vi "plotAnkleTraj.vi"(4 "AnkleTraj_Prev":dbl[][](array[numeric]), 5 "AnkleTraj_history":dbl[][](array[numeric]), 6 "Init?":bool, 8 "error in (no error)":errorcluster, 9 "PreviousPlotNum":i32, 10 "3D graph in":refnum<k7>) -> (0 "error out":errorcluster, 1 "LastPlotNum":i32=1, 2 "3D graph out":refnum<k7>)   [LabVIEW 2016]
uses:
  <vilib>/Platform/NI_3dgraph.lvlib
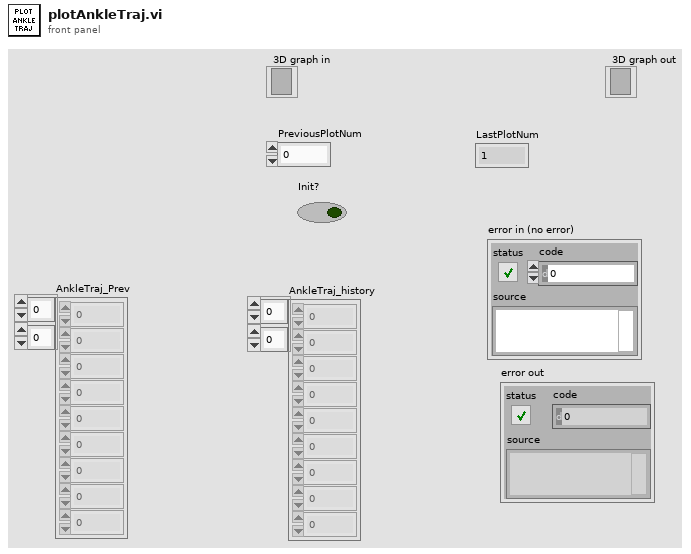
[diagram p1: front panel]
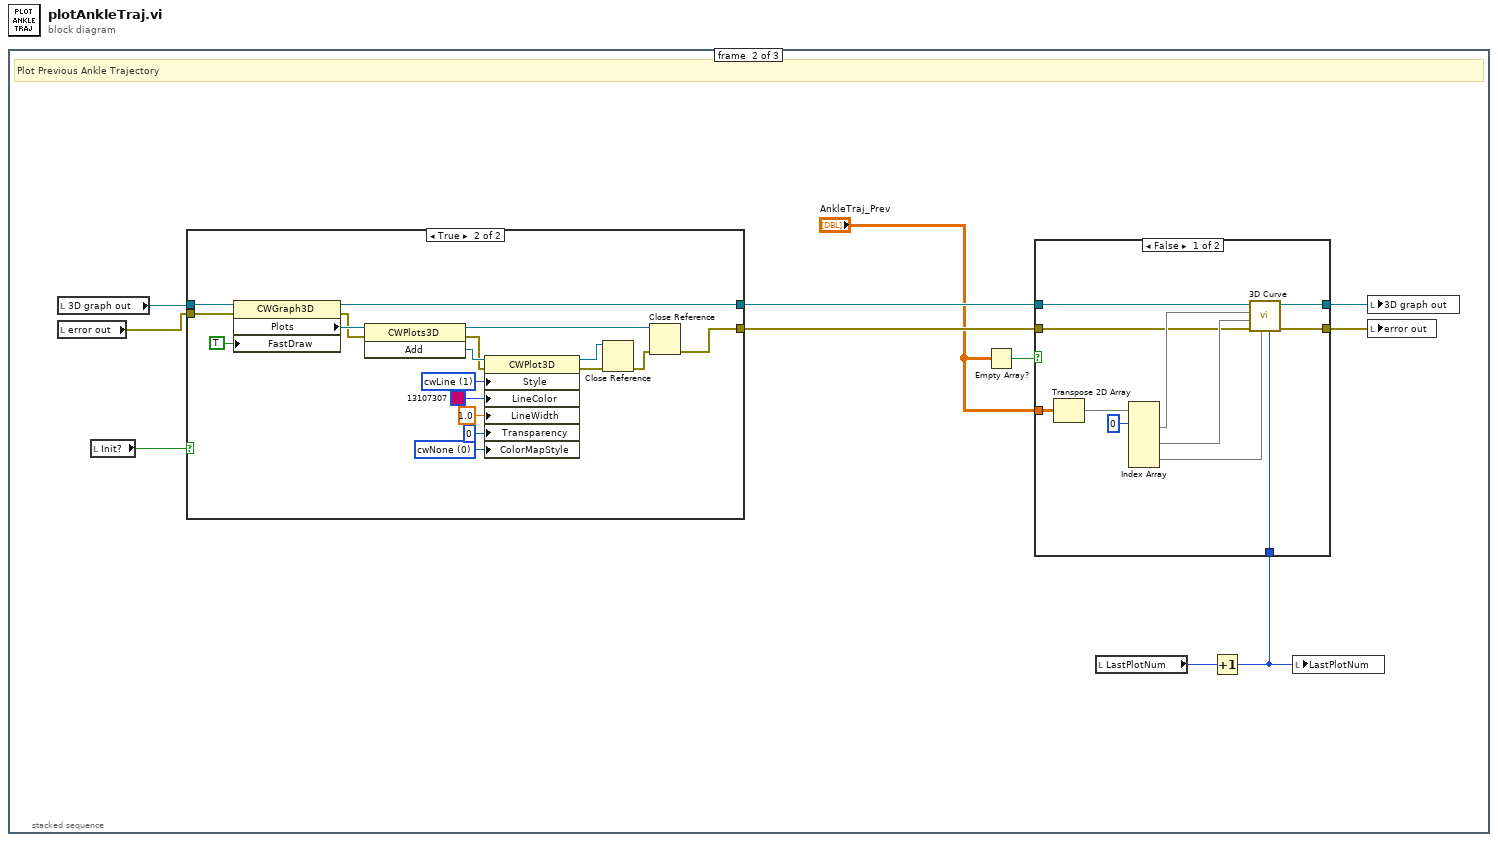
[diagram p0: block diagram]
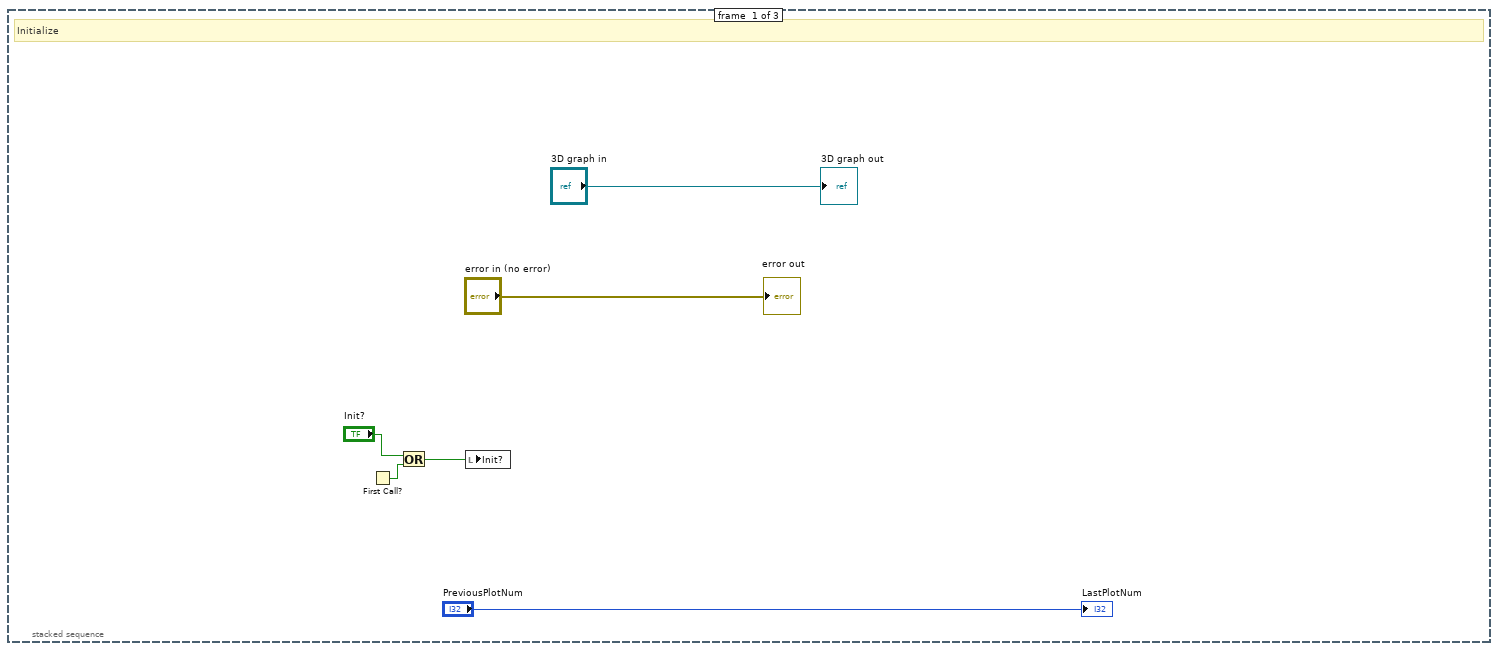
[diagram p2: hidden frame]
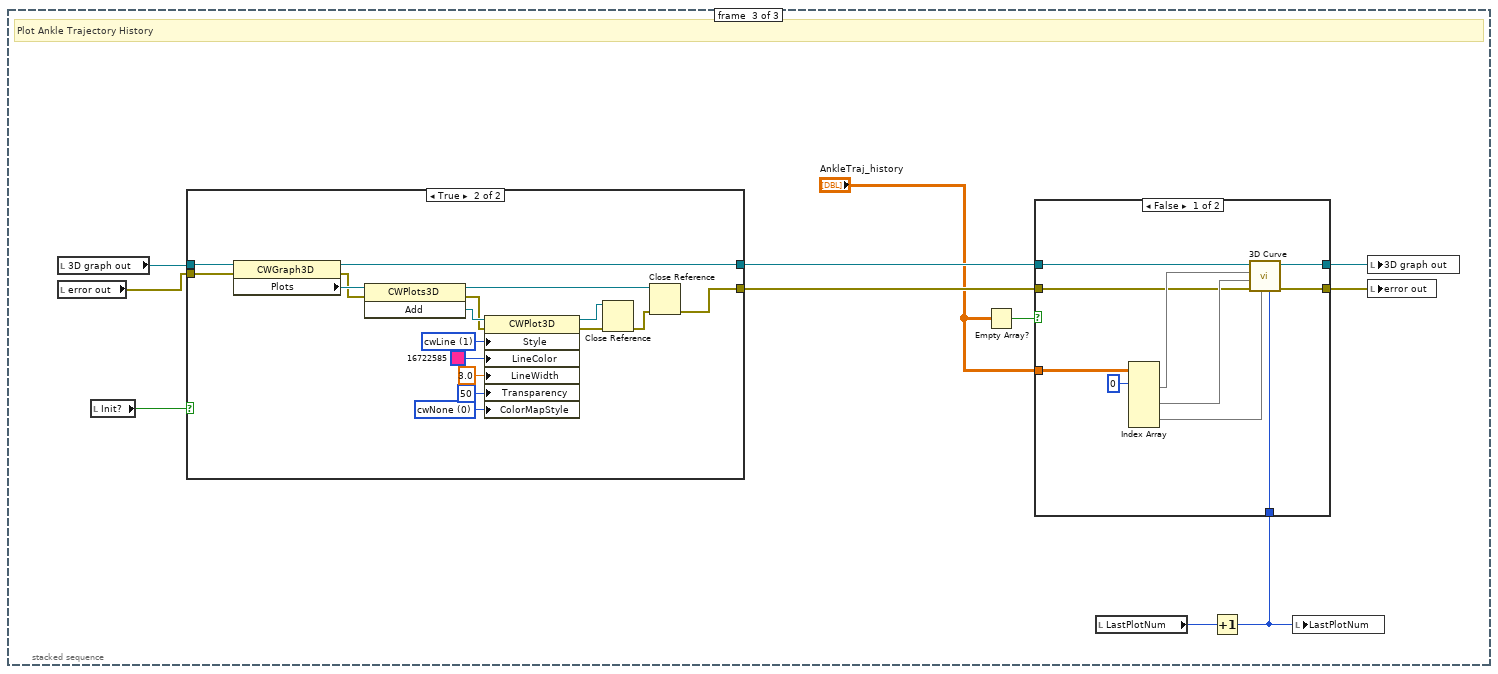
[diagram p5: hidden frame]
diagram:
  n1 = stacked-sequence {
    frame #0 {
      # "Initialize"
      n2 = First Call?() -> (First Call?: T/F=w3:bool)
      n3 = Or(x="Init?", y=w3) -> (x .or. y?=w1:bool)
      n4 = local write "Init?"(w1) -> ()
      "LastPlotNum" <- "PreviousPlotNum"
      "error out" <- "error in (no error)"
      "3D graph out" <- "3D graph in"
    }
    frame #1 {
      # "Plot Previous Ankle Trajectory"
      n5 = local read "3D graph out"() -> (w9:refnum<k7>)
      n6 = local read "error out"() -> (w8:errorcluster)
      n7 = local read "Init?"() -> (w7:bool)
      n8 = case shown="True" w7 {
        tunnel: w8 -> [w31 w43]
        tunnel: w9 -> [w32 w40]
        tunnel: [w32 w39] -> w17
        tunnel: [w31 w34] -> w16
        frame False {
        }
        frame True {
          w37 = 0 items=["cwNone", "cwShaded", "cwColorSpectrum", "cwGrayScale", "cwCustom"] ("ColorMapStyle")
          w50 = 1 items=["cwLine"=1, "cwPoint"=2, "cwLinePoint"=3, "cwHiddenLine"=4, "cwSurface"=5, "cwSurfaceLine"=6, "cwSurfaceNormal"=7, "cwContourLine"=8, "cwSurfaceContour"=9] ("Style")
          n9 = property class="CWGraph3D"(reference=w40, error in=w43, "FastDraw"=TRUE) -> (reference out=w39:refnum<k7>, error out=w47:errorcluster, "Plots"=w48:refnum<k7>)
          n10 = invoke class="CWPlots3D" method="Add"(reference=w48, error in=w47) -> (reference out=w46:refnum<k7>, error out=w36:errorcluster, "Add"=w49:refnum<k7>)  [unwired: 1 in]
          n11 = property class="CWPlot3D"(reference=w49, error in=w36, "Style"=w50, "LineColor"=u32 13107307, "LineWidth"=1.0, "Transparency"=0, "ColorMapStyle"=w37) -> (reference out=w44:refnum<k7>, error out=w45:errorcluster)
          n12 = Close Reference(reference=w44, error in (no error)=w45) -> (error out=w35:errorcluster)
          n13 = Close Reference(reference=w46, error in (no error)=w35) -> (error out=w34:errorcluster)
        }
      }
      n14 = Empty Array?(array="AnkleTraj_Prev") -> (empty?=w15:bool)
      n15 = local read "LastPlotNum"() -> (w13:i32)
      n16 = Increment(x=w13) -> (x+1=w12:i32)
      n17 = case shown="False" w15 {
        tunnel: "AnkleTraj_Prev" -> [w28 _]
        tunnel: [w22 w30] -> w11
        tunnel: w17 -> [w21 w30]
        tunnel: w12 -> [w20 _]
        tunnel: w16 -> [w19 w29]
        tunnel: [w18 w29] -> w10
        frame False {
          n18 = Transpose 2D Array(2D array=w28) -> (transposed array=w23:dbl[][])
          n19 = Index Array(array=w23, index (row) #1=0 ("index (row)")) -> (element #1=w25:dbl[], element #2=w26:dbl[], element #3=w27:dbl[])  [unwired: 5 in]
          n20 = call <vilib>:"3D Curve.vi"("plot number (1)"=w20, "z vector"=w27, "error in (no error)"=w19, "y vector"=w26, "x vector"=w25, "3D graph"=w21) -> ("error out"=w18:errorcluster, "3D graph out"=w22:refnum<k7>)  [unwired: 4 in]
        }
        frame True {
        }
      }
      n21 = local write "LastPlotNum"(w12) -> ()
      n22 = local write "3D graph out"(w11) -> ()
      n23 = local write "error out"(w10) -> ()
    }
    frame #2 {
      # "Plot Ankle Trajectory History"
      n24 = local read "3D graph out"() -> (w53:refnum<k7>)
      n25 = local read "error out"() -> (w52:errorcluster)
      n26 = local read "Init?"() -> (w51:bool)
      n27 = case shown="True" w51 {
        tunnel: w52 -> [w74 w85]
        tunnel: w53 -> [w75 w82]
        tunnel: [w75 w81] -> w61
        tunnel: [w74 w76] -> w60
        frame False {
        }
        frame True {
          w79 = 0 items=["cwNone", "cwShaded", "cwColorSpectrum", "cwGrayScale", "cwCustom"] ("ColorMapStyle")
          w92 = 1 items=["cwLine"=1, "cwPoint"=2, "cwLinePoint"=3, "cwHiddenLine"=4, "cwSurface"=5, "cwSurfaceLine"=6, "cwSurfaceNormal"=7, "cwContourLine"=8, "cwSurfaceContour"=9] ("Style")
          n28 = property class="CWGraph3D"(reference=w82, error in=w85) -> (reference out=w81:refnum<k7>, error out=w89:errorcluster, "Plots"=w90:refnum<k7>)
          n29 = invoke class="CWPlots3D" method="Add"(reference=w90, error in=w89) -> (reference out=w88:refnum<k7>, error out=w78:errorcluster, "Add"=w91:refnum<k7>)  [unwired: 1 in]
          n30 = property class="CWPlot3D"(reference=w91, error in=w78, "Style"=w92, "LineColor"=u32 16722585, "LineWidth"=3.0, "Transparency"=50, "ColorMapStyle"=w79) -> (reference out=w86:refnum<k7>, error out=w87:errorcluster)
          n31 = Close Reference(reference=w86, error in (no error)=w87) -> (error out=w77:errorcluster)
          n32 = Close Reference(reference=w88, error in (no error)=w77) -> (error out=w76:errorcluster)
        }
      }
      n33 = Empty Array?(array="AnkleTraj_history") -> (empty?=w59:bool)
      n34 = local read "LastPlotNum"() -> (w57:i32)
      n35 = Increment(x=w57) -> (x+1=w56:i32)
      n36 = case shown="False" w59 {
        tunnel: "AnkleTraj_history" -> [w62 _]
        tunnel: [w67 w73] -> w55
        tunnel: w61 -> [w66 w73]
        tunnel: w56 -> [w65 _]
        tunnel: w60 -> [w64 w72]
        tunnel: [w63 w72] -> w54
        frame False {
          n37 = Index Array(array=w62, index (row) #1=0 ("index (row)")) -> (element #1=w69:dbl[], element #2=w70:dbl[], element #3=w71:dbl[])  [unwired: 5 in]
          n38 = call <vilib>:"3D Curve.vi"("plot number (1)"=w65, "z vector"=w71, "error in (no error)"=w64, "y vector"=w70, "x vector"=w69, "3D graph"=w66) -> ("error out"=w63:errorcluster, "3D graph out"=w67:refnum<k7>)  [unwired: 4 in]
        }
        frame True {
        }
      }
      n39 = local write "LastPlotNum"(w56) -> ()
      n40 = local write "3D graph out"(w55) -> ()
      n41 = local write "error out"(w54) -> ()
    }
  }
